vi "Sun Lat-Lon.vi"(8 "error in (no error)":errorcluster, 11 "Lat/Lon string":string) -> (0 "error out":errorcluster, 1 "Minutes":i32, 2 "Degrees":i32, 3 "Converted Position":dbl, 5 "Direction":string)   [LabVIEW 2018]
doc: "Conversion of the <b>Lat/Lon string</b> in Degree/Minute format used on timeanddate.com to numerical values: <b>Converted position</b> returns decimal form, <b>Degrees</b> and <b>Minutes</b> return integer degree and minute values. \n\nReturn Error code 5005 in case of problems."
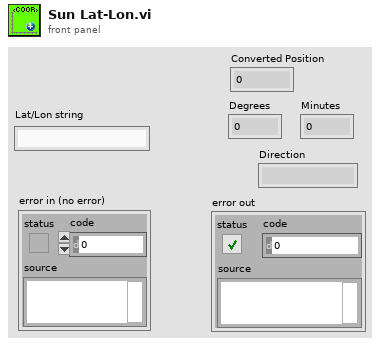
[diagram p1: front panel]
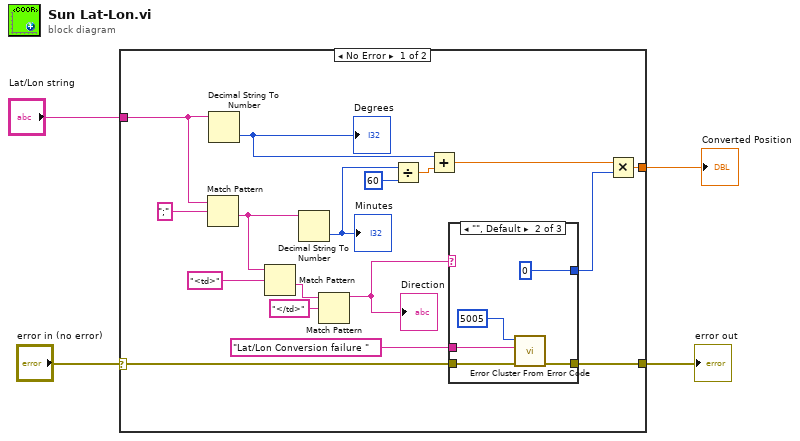
[diagram p0: block diagram]
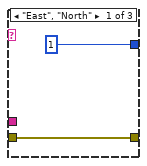
[diagram p2: hidden frame]
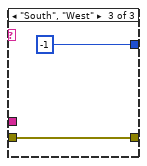
[diagram p3: hidden frame]
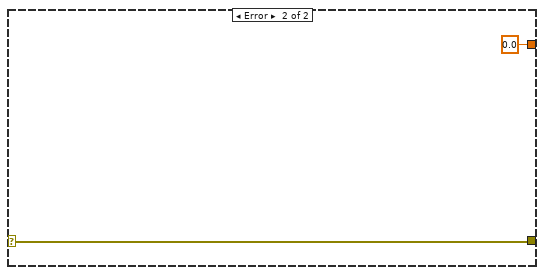
[diagram p4: hidden frame]
diagram:
  n1 = case shown="No Error" "error in (no error)" {
    selector: "error in (no error)" -> [w9 w32]
    tunnel: [w21 0.0] -> w4
    tunnel: "Lat/Lon string" -> [w12 _]
    tunnel: [w8 w32] -> w1
    frame No Error {
      n2 = Match Pattern(string=w12, regular expression=";") -> (after substring=w14:string)  [unwired: 1 in, 3 out]
      n3 = Decimal String To Number(string=w12) -> (number=w18:i32)  [unwired: 2 in, 1 out]
      "Degrees" <- w18
      n4 = Match Pattern(string=w14, regular expression="<td>") -> (after substring=w7:string)  [unwired: 1 in, 3 out]
      n5 = Decimal String To Number(string=w14) -> (number=w15:i32)  [unwired: 2 in, 1 out]
      "Minutes" <- w15
      n6 = Match Pattern(string=w7, regular expression="</td>") -> (before substring=w5:string)  [unwired: 1 in, 3 out]
      "Direction" <- w5
      n7 = Divide(x=w15, y=60) -> (x/y=w17:dbl)
      n8 = Add(x=w18, y=w17) -> (x+y=w19:dbl)
      n9 = case shown="\"\", Default" w5 {
        tunnel: [1 0 -1] -> w20
        tunnel: "Lat/Lon Conversion failure " -> [_ w26 _]
        tunnel: [w22 w25 w29] -> w8
        tunnel: w9 -> [w22 w24 w29]
        frame "East", "North" {
        }
        frame "", Default {
          n10 = call <vilib>:"Error Cluster From Error Code.vi"("error in (no error)"=w24, "error message (\"\")"=w26, "error code (0)"=5005) -> ("error out"=w25:errorcluster)  [unwired: 6 in]
        }
        frame "South", "West" {
        }
      }
      n11 = Multiply(x=w19, y=w20) -> (x*y=w21:dbl)
    }
    frame Error {
    }
  }
  "Converted Position" <- w4
  "error out" <- w1
